vi "constructor.vi"(8 "error in (no error)":errorcluster, 9 "machine name":string, 10 "Camera":string) -> (0 "error out":errorcluster, 3 "NetworkCamera out":refnum<class "NetworkCamera.lvclass">)   [LabVIEW 2011, in "Hardware.lvlib" / "HWControllers.lvlib" / "NetworkCamera.lvclass"]
uses:
  NetworkCamera.lvclass
  NetworkWinX32/NetworkWinX32.lvclass
  NetworkPixelfly/NetworkPixelfly.lvclass
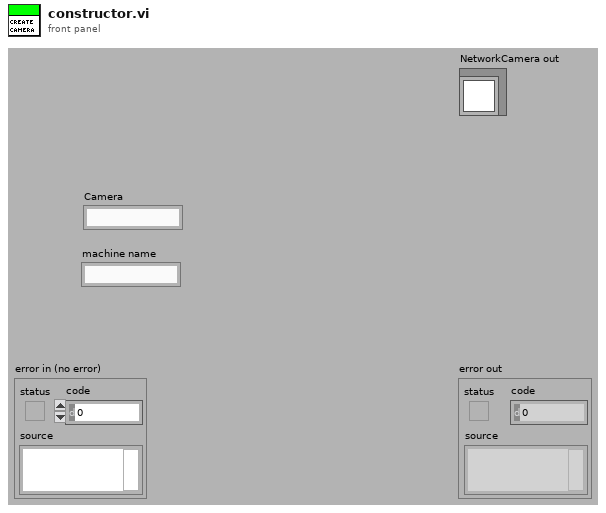
[diagram p1: front panel]
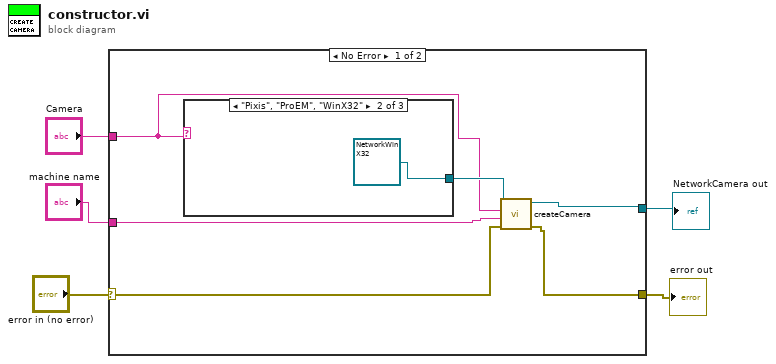
[diagram p0: block diagram]
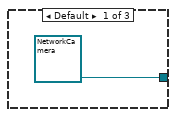
[diagram p2: hidden frame]
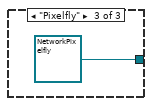
[diagram p3: hidden frame]
diagram:
  n1 = case shown="No Error" "error in (no error)" {
    selector: "error in (no error)" -> [w9 w15]
    tunnel: [w8 w15] -> w4
    tunnel: [w11 _] -> w3
    tunnel: "Camera" -> [w6 _]
    tunnel: "machine name" -> [w7 _]
    frame No Error {
      n2 = case shown="\"Pixis\", \"ProEM\", \"WinX32\"" w6 {
        tunnel: [refnum<class "NetworkCamera.lvclass"> refnum ("Hardware:HWControllers.lvlib:NetworkCamera.lvclass") refnum<class "NetworkWinX32.lvclass"> refnum ("Hardware:HWControllers.lvlib:NetworkWinX32.lvclass") refnum<class "NetworkPixelfly.lvclass"> refnum ("Hardware:HWControllers.lvlib:NetworkPixelfly.lvclass")] -> w10
        frame Default {
        }
        frame "Pixis", "ProEM", "WinX32" {
        }
        frame "Pixelfly" {
        }
      }
      n3 = call-dynamic "createCamera.vi"("error in (no error)"=w9, "machine name"=w7, "Camera"=w6, "NetworkCamera in"=w10) -> ("error out"=w8:errorcluster, "NetworkCamera out"=w11:refnum<class "NetworkCamera.lvclass">)  [unwired: 6 in]
    }
    frame Error {
    }
  }
  "error out" <- w4
  "NetworkCamera out" <- w3
